vi "createMissionWaypoints.vi"(8 "error in (no error)":errorcluster, 11 "PassBuoys in":refnum<class "PassBuoys.lvclass">) -> (0 "error out":errorcluster, 3 "PassBuoys out":refnum<class "PassBuoys.lvclass">)   [LabVIEW 2011, in "PassBuoys.lvclass"]
doc: "Creates three waypoint objects for the mission, and puts them in the queue. The first waypoint is in front of the two buoys. The second is at their midpoint. The third is just past them. No sail zones are positioned on the two buoys. The distances and tolerances are set on the front panel, in meters. (The third waypoint has double the tolerance of the first two)."
uses:
  PassBuoys.lvclass
  Waypoint/Waypoint.lvclass
  2 Globals/2 Global.vi
panel:
  in  "Distance from Center":dbl=10.0
  in  "Tolerance (meters)":dbl=3.0
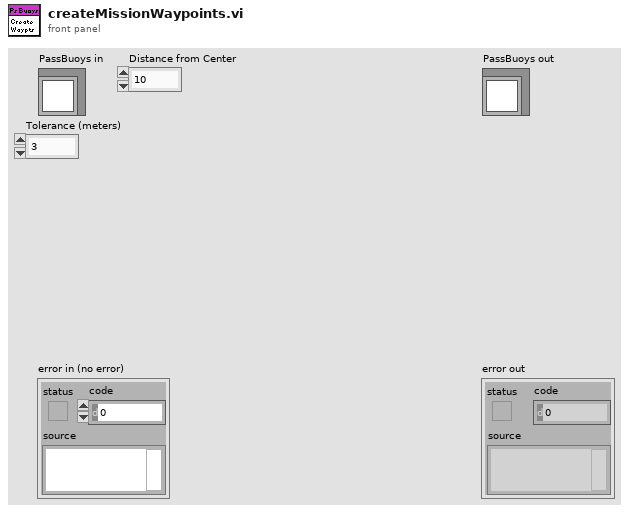
[diagram p1: front panel]
types:
  T1 = typedef "UTM Location.ctl" = cluster{"UTM Zone":dbl, "Hemisphere":enum16{"North", "South"}, "East":dbl, "North":dbl}
  T2 = typedef "UTM Circle.ctl" = cluster{"UTM Zone":dbl, "Hemisphere":enum16{"North", "South"}, "East":dbl, "North":dbl, "Radius":dbl}
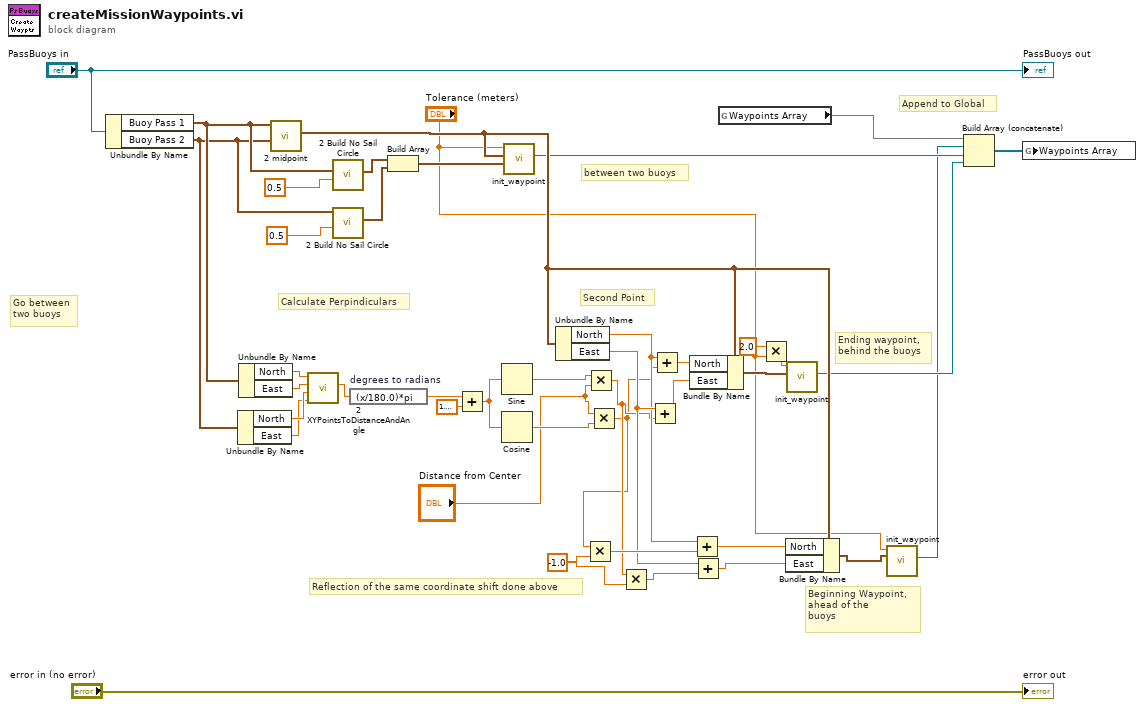
[diagram p0: block diagram]
diagram:
  w1 = -1.0 ("y")
  # "Reflection of the same coordinate shift done above"
  # "between two buoys"
  # "Calculate Perpindiculars"
  # "Ending waypoint,\nbehind the buoys"
  # "Beginning Waypoint,\nahead of the\nbuoys"
  # "Second Point"
  # "Go between\ntwo buoys"
  # "Append to Global"
  n1 = Unbundle By Name("PassBuoys in") -> ("Buoy Pass 1"=w13:T1, "Buoy Pass 2"=w12:T1)
  n2 = Unbundle By Name(w12) -> ("North"=w33:dbl, "East"=w32:dbl)
  n3 = Unbundle By Name(w13) -> ("North"=w35:dbl, "East"=w34:dbl)
  n4 = call "2 midpoint.vi"("UTM 2"=w12, "UTM 1"=w13) -> ("Midpoint"=w19:T1)  [unwired: 8 in, 1 out]
  n5 = call "2 XYPointsToDistanceAndAngle.vi"("East 2"=w32, "North 2"=w33, "East 1"=w34, "North 1"=w35) -> ("Angle Diff"=w6:dbl)  [unwired: 6 in, 1 out]
  n6 = call "2 Build No Sail Circle.vi"("Radius"=0.5, "UTM Location"=w13) -> ("UTM Circle"=w41:T2)  [unwired: 9 in]
  n7 = call "2 Build No Sail Circle.vi"("Radius"=0.5, "UTM Location"=w12) -> ("UTM Circle"=w39:T2)  [unwired: 9 in]
  n8 = expression code="(x/180.0)*pi" "degrees to radians"(w6) -> (w7:dbl)
  n9 = Build Array(w41, w39) -> (w42:T2[])
  n10 = Add(x=w7, y=1.5707963267948966) -> (x+y=w31:dbl)
  n11 = Sine(x=w31) -> (sin(x)=w27:dbl)
  n12 = Cosine(x=w31) -> (cos(x)=w26:dbl)
  n13 = call "init_waypoint.vi"("No Sail Circles"=w42, "Coords"=w19, "Tolerance (m)"="Tolerance (meters)") -> ("Waypoint Out"=w16:refnum<class "Waypoint.lvclass">)  [unwired: 8 in]
  n14 = Unbundle By Name(w19) -> ("North"=w22:dbl, "East"=w23:dbl)
  n15 = Multiply(x=w27, y="Distance from Center") -> (x*y=w10:dbl)
  n16 = Multiply(x="Distance from Center", y=w26) -> (x*y=w9:dbl)
  n17 = Multiply(x=w9, y=w1) -> (x*y=w24:dbl)
  n18 = Multiply(x=w10, y=w1) -> (x*y=w25:dbl)
  n19 = Add(x=w23, y=w10) -> (x+y=w30:dbl)
  n20 = Add(x=w22, y=w9) -> (x+y=w29:dbl)
  n21 = Bundle By Name(cluster=w19, "North"=w29, "East"=w30) -> (w28:T1)
  n22 = Add(x=w22, y=w24) -> (x+y=w21:dbl)
  n23 = Add(x=w23, y=w25) -> (x+y=w20:dbl)
  n24 = global read "2 Global.vi" "Waypoints Array"() -> (w37)
  n25 = Multiply(x=2.0, y="Tolerance (meters)") -> (x*y=w5:dbl)
  n26 = Bundle By Name(cluster=w19, "North"=w21, "East"=w20) -> (w18:T1)
  n27 = call "init_waypoint.vi"("Coords"=w28, "Tolerance (m)"=w5) -> ("Waypoint Out"=w17:refnum<class "Waypoint.lvclass">)  [unwired: 9 in]
  n28 = call "init_waypoint.vi"("Coords"=w18, "Tolerance (m)"="Tolerance (meters)") -> ("Waypoint Out"=w15:refnum<class "Waypoint.lvclass">)  [unwired: 9 in]
  n29 = Build Array (concatenate)(w37, w15, w16, w17) -> (w36:refnum<class "Waypoint.lvclass">[])
  n30 = global write "2 Global.vi" "Waypoints Array"(w36) -> ()
  "error out" <- "error in (no error)"
  "PassBuoys out" <- "PassBuoys in"
